vi "StartDAQ notifier.vi"(4 "error in (no error)":errorcluster, 5 "wait for DAQ? (F)":bool) -> (0 "error out":errorcluster)   [LabVIEW 2020]
doc: "Sends <B>Start</B> notifier to DAQ thread to begin measurement."
uses:
  DAQ Engine VIs/PXI Globals.vi
panel:
  out "x > 0?":bool
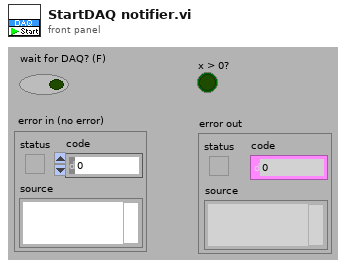
[diagram p1: front panel]
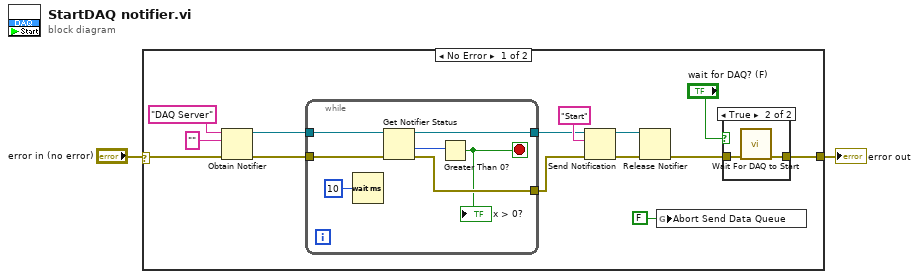
[diagram p0: block diagram]
diagram:
  n1 = case shown="No Error" "error in (no error)" {
    selector: "error in (no error)" -> [w8 w27]
    tunnel: [w4 w27] -> w1
    frame No Error {
      n2 = Obtain Notifier(name (unnamed)="DAQ Server", notification data type="", error in (no error)=w8) -> (notifier out=w12:refnum<notifier>, error out=w13:errorcluster)  [unwired: 1 in, 1 out]
      n3 = while {
        tunnel: w12 -> [w25]
        tunnel: w13 -> [w24]
        tunnel: [w22] -> w9
        tunnel: [w21] -> w7
        stop <- w20 stop-if-true
        n4 = Wait (ms)(milliseconds to wait=10) -> ()  [unwired: 1 out]
        n5 = Get Notifier Status(notifier=w25, error in (no error)=w24) -> (notifier out=w22:refnum<notifier>, # waiting=w23:i32, error out=w21:errorcluster)  [unwired: 2 out]
        n6 = Greater Than 0?(x=w23) -> (x > 0?=w20:bool)
        "x > 0?" <- w20
      }
      n7 = Send Notification(notification="Start", notifier=w9, error in (no error)=w7) -> (notifier out=w11:refnum<notifier>, error out=w10:errorcluster)
      n8 = Release Notifier(notifier=w11, error in (no error)=w10) -> (error out=w5:errorcluster)  [unwired: 1 in, 2 out]
      n9 = global write "PXI Globals.vi" "Abort Send Data Queue"(FALSE ("Abort Send Data Queue")) -> ()
      n10 = case shown="True" "wait for DAQ? (F)" {
        tunnel: w5 -> [w17 w19]
        tunnel: [w17 w18] -> w4
        frame False {
        }
        frame True {
          n11 = call "Wait For DAQ to Start.vi"("error in (no error)"=w19) -> ("error out"=w18:errorcluster)  [unwired: 10 in]
        }
      }
    }
    frame Error {
    }
  }
  "error out" <- w1
